vi "Подключение (SubVI) (2).vi"(8 "error in":errorcluster, 11 "UnicornParam":T1={"ReadIntParam"=FALSE, "ReadDescrParam"=FALSE, "ReadFloatParam"=FALSE, "debug"=FALSE, "ReadJSON"=FALSE, "IP_address"="", "N_attempts"=0, "type_con"=enum."Serial", "MB_address"=0, "VISA"="", "connection ID"=refnum, "nameDevices"="", "timeout"=0, "port"=0, "type_version"="", "baud_rate"=0, "VersionControl"=TRUE, "TCP_conn"=TRUE, "WindowSize"=700}) -> (0 "error out":errorcluster, 1 "JSONStruct":T2={"NumParam"={"NTelem"=201, "NInt"=16, "NFloat"=10, "NTable"=2}, "ParamInt"=[], "Telemetry"=[], "Table"=[], "ParamFloat"=[]}, 2 "IntFloat":cluster{"ArrayInt":i32[], "ArrayFloat":sgl[]}, 3 "Parameter Out":T1={"ReadIntParam"=FALSE, "ReadDescrParam"=FALSE, "ReadFloatParam"=FALSE, "debug"=FALSE, "ReadJSON"=FALSE, "IP_address"="", "N_attempts"=0, "type_con"=enum."Serial", "MB_address"=0, "VISA"="", "connection ID"=refnum, "nameDevices"="", "timeout"=0, "port"=0, "type_version"="", "baud_rate"=0, "VersionControl"=TRUE, "TCP_conn"=TRUE, "WindowSize"=700}, 4 "TableParamName":string[][](array[string]), 5 "NParam":cluster{"NTelem":i32, "NInt":i32, "NFloat":i32}, 7 "NoConnection":bool)   [LabVIEW 2017, in "Unicorn Library.lvlib"]
uses:
  Unicorn Library.lvlib
  Control/unicorn_JSON.ctl
  Control/unicorn_Telemetry.ctl
  Control/unicorn_ParamInt.ctl
  Control/unicorn_Table.ctl
  Control/unicorn_ParamFloat.ctl
  Control/unicorn_conn.ctl
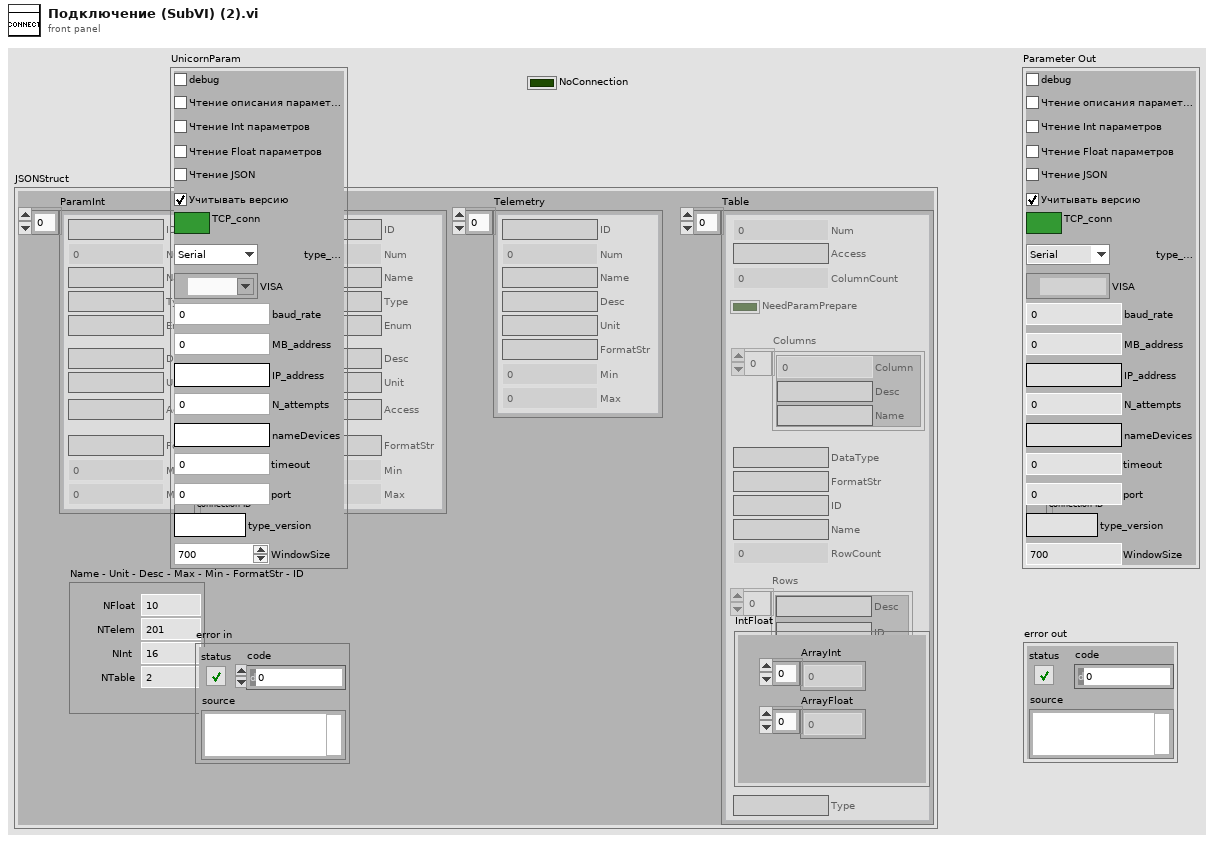
[diagram p1: front panel]
types:
  T1 = typedef "Unicorn Library.lvlib/unicorn_conn.ctl" = cluster{"ReadIntParam":bool, "ReadDescrParam":bool, "ReadFloatParam":bool, "debug":bool, "ReadJSON":bool, "IP_address":string, "N_attempts":i32, "type_con":enum16{"Serial", "TCP"}, "MB_address":i32, "VISA":refnum<visa-resource-name>, "connection ID":refnum<k5>, "nameDevices":string, "timeout":i32, "port":u16, "type_version":string, "baud_rate":u32, "VersionControl":bool, "TCP_conn":bool, "WindowSize":i32}
  T2 = typedef "Unicorn Library.lvlib/unicorn_JSON.ctl" = cluster{"NumParam":cluster{"NTelem":i32, "NInt":i32, "NFloat":i32, "NTable":i32}, "ParamInt":T3, "Telemetry":T4, "Table":T5, "ParamFloat":T6}
  T3 = typedef "Unicorn Library.lvlib/unicorn_ParamInt.ctl" = cluster{"ID":string, "Num":i32, "Name":string, "Type":string, "Enum":string, "Desc":string, "Unit":string, "Access":string, "FormatStr":string, "Min":i32, "Max":i32}[]
  T4 = typedef "Unicorn Library.lvlib/unicorn_Telemetry.ctl" = cluster{"ID":string, "Num":i32, "Name":string, "Desc":string, "Unit":string, "FormatStr":string, "Min":i32, "Max":i32}[]
  T5 = typedef "Unicorn Library.lvlib/unicorn_Table.ctl" = cluster{"Num":i32, "Access":string, "ColumnCount":i32, "NeedParamPrepare":bool, "Columns":cluster{"Column":i32, "Desc":string, "Name":string}[], "DataType":string, "FormatStr":string, "ID":string, "Name":string, "RowCount":i32, "Rows":cluster{"Desc":string, "ID":string, "Max":i32, "Min":i32, "Name":string, "Row":i32, "Unit":string}[], "Type":string}[]
  T6 = typedef "Unicorn Library.lvlib/unicorn_ParamFloat.ctl" = cluster{"ID":string, "Num":i32, "Name":string, "Type":string, "Enum":string, "Desc":string, "Unit":string, "Access":string, "FormatStr":string, "Min":i32, "Max":i32}[]
  T7 = typedef "Unicorn Library.lvlib/unicorn_Param.ctl" = cluster{"conParam":T1, "Param":T2}
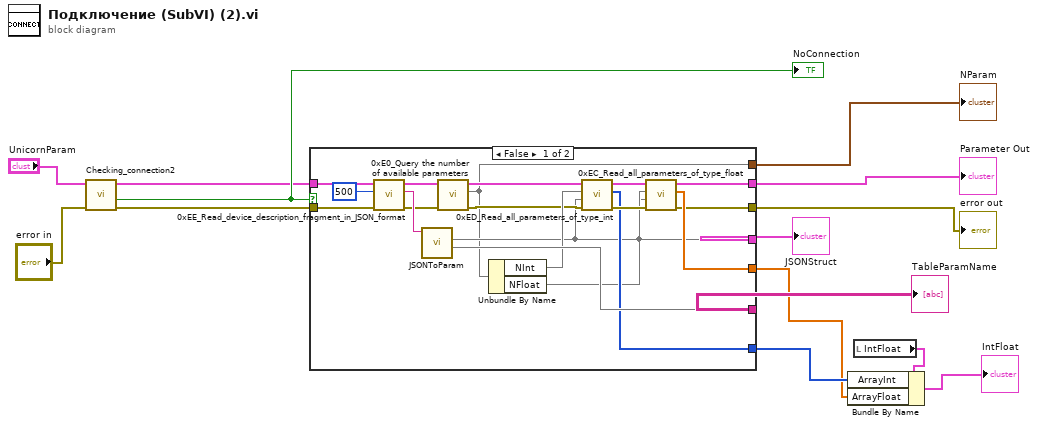
[diagram p0: block diagram]
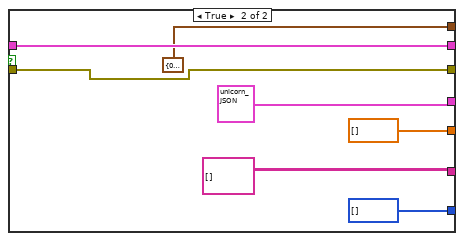
[diagram p2: hidden frame]
diagram:
  n1 = call "Checking_connection2.vi"("error in"="error in", "paramUnicornIn"="UnicornParam") -> ("error out"=w9:errorcluster, "NoConnection"=w11:bool, "paramUnicorn"=w8:T7)  [unwired: 6 in, 1 out]
  "NoConnection" <- w11
  n2 = case shown="False" w11 {
    tunnel: w8 -> [w33 w40]
    tunnel: w9 -> [w31 w34]
    tunnel: [w21 w40] -> w10
    tunnel: [w17 T2 {"NumParam"={"NTelem"=201, "NInt"=16, "NFloat"=10, "NTable"=2}, "ParamInt"=[{"ID"="Режим работы", "Num"=0, "Name"="", "Type"="", "Enum"="", "Desc"="", "Unit"="", "Access"="", "FormatStr"="", "Min"=0, "Max"=0}, {"ID"="", "Num"=0, "Name"="", "Type"="", "Enum"="", "Desc"="", "Unit"="", "Access"="", "FormatStr"="", "Min"=0, "Max"=0}, {"ID"="", "Num"=0, "Name"="", "Type"="", "Enum"="", "Desc"="", "Unit"="", "Access"="", "FormatStr"="", "Min"=0, "Max"=0}, {"ID"="", "Num"=0, "Name"="", "Type"="", "Enum"="", "Desc"="", "Unit"="", "Access"="", "FormatStr"="", "Min"=0, "Max"=0}, {"ID"="", "Num"=0, "Name"="", "Type"="", "Enum"="", "Desc"="", "Unit"="", "Access"="", "FormatStr"="", "Min"=0, "Max"=0}, {"ID"="", "Num"=0, "Name"="", "Type"="", "Enum"="", "Desc"="", "Unit"="", "Access"="", "FormatStr"="", "Min"=0, "Max"=0}, {"ID"="ModeWork", "Num"=0, "Name"="", "Type"="", "Enum"="", "Desc"="", "Unit"="", "Access"="", "FormatStr"="", "Min"=0, "Max"=0}], "Telemetry"=[], "Table"=[], "ParamFloat"=[]} ("JSONStruct")] -> w12
    tunnel: [w29 string[][] [] ("TableParamName")] -> w13
    tunnel: [w20 sgl[] [] ("ArrayFloat")] -> w5
    tunnel: [w19 i32[] [] ("ArrayInt")] -> w6
    tunnel: [w16 cluster{"NTelem":i32, "NInt":i32, "NFloat":i32} {"NTelem"=0, "NInt"=0, "NFloat"=0} ("NParam")] -> w14
    tunnel: [w15 w34] -> w2
    frame False {
      n3 = call "0xEE_Read_device_description_fragment_in_JSON_format.vi"("error in"=w31, "Макс размер"=500, "paramUnicorn 2"=w33) -> ("error out"=w24:errorcluster, "JSONStr"=w30:string, "paramUnicorn"=w28:T7)  [unwired: 6 in]
      n4 = call "JSONToParam.vi"("paramUnicornIn"=w30) -> (1:w29, 2:w17)  [unwired: 7 in, 2 out]
      n5 = call "0xE0_Query the number of available parameters.vi"("error in"=w24, "paramUnicorn"=w28) -> ("error out"=w25:errorcluster, 2:w16, "paramUnicorn out"=w27:T7)  [unwired: 5 in, 2 out]
      n6 = Unbundle By Name(w16) -> ("NInt"=w26, "NFloat"=w18)
      n7 = call "0xED_Read_all_parameters_of_type_int.vi"("error in"=w25, 9:w17, 10:w26, "paramUnicorn"=w27) -> ("error out"=w22:errorcluster, "ArrayInt"=w19:i32[], "paramUnicorn 2"=w23:T7)  [unwired: 4 in, 1 out]
      n8 = call "0xEC_Read_all_parameters_of_type_float.vi"("error in"=w22, 9:w17, 10:w18, "paramUnicorn"=w23) -> ("error out"=w15:errorcluster, "ArrayFloat"=w20:sgl[], "paramUnicorn 2"=w21:T7)  [unwired: 4 in, 1 out]
    }
    frame True {
    }
  }
  "NParam" <- w14
  "TableParamName" <- w13
  "JSONStruct" <- w12
  "Parameter Out" <- w10
  "error out" <- w2
  n9 = local read "IntFloat"() -> (w3:cluster{"ArrayInt":i32[], "ArrayFloat":sgl[]})
  n10 = Bundle By Name(cluster=w3, "ArrayInt"=w6, "ArrayFloat"=w5) -> (→"IntFloat":cluster{"ArrayInt":i32[], "ArrayFloat":sgl[]})
